vi "Write Str Refnum.vi"(8 "error in (no error)":errorcluster, 10 "Str Refnum":refnum<vi>, 11 "Dialog.lvclass in":refnum<class "Dialog.lvclass">) -> (0 "error out":errorcluster, 3 "Dialog.lvclass out":refnum<class "Dialog.lvclass">)   [LabVIEW 2012, in "Dialog.lvlib" / "Dialog.lvclass"]
uses:
  Dialog.lvclass
  Dialog.lvclass/Dialog.ctl
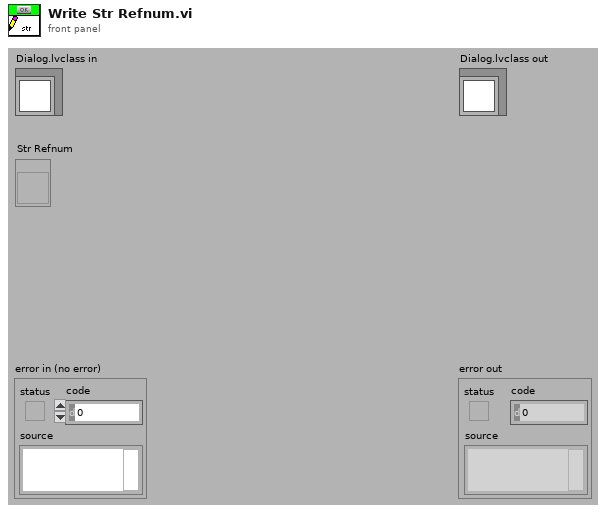
[diagram p1: front panel]
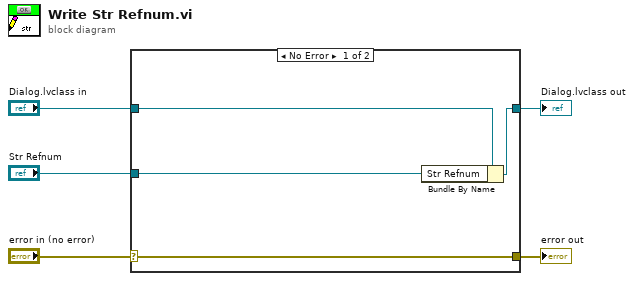
[diagram p0: block diagram]
diagram:
  n1 = case shown="No Error" "error in (no error)" {
    selector: "error in (no error)" -> [w9 w10]
    tunnel: [w9 w10] -> w4
    tunnel: [w7 w11] -> w2
    tunnel: "Dialog.lvclass in" -> [w8 w11]
    tunnel: "Str Refnum" -> [w6 _]
    frame No Error {
      n2 = Bundle By Name(cluster=w8, "Str Refnum"=w6) -> (w7:refnum<class "Dialog.lvclass">)
    }
    frame Error {
    }
  }
  "error out" <- w4
  "Dialog.lvclass out" <- w2
